vi "Unpack User Menu Selection.vi"(11 "UserMenuSelectionMsg In":refnum<class "UserMenuSelectionMsg.lvclass">) -> (0 "Item Path":string, 1 "Item Tag":string, 2 "Time":u32, 3 "MenuRef":refnum<k9>)   [LabVIEW 2015, in "ActorEvents.lvlib" / "UserMenuSelectionMsg.lvclass"]
doc: "<License>\nCopyright © 2017 Composed Systems, LLC | All rights reserved\nwww.composed.io\n\nAuthor: Ethan Stern <ethan.stern@composed.io>\n\nThis software is provided \"AS IS\" WITHOUT WARRANTIES, either express or implied, AND IS FOR EDUCATIONAL PURPOSES ONLY.\n</License>"
uses:
  UserMenuSelectionMsg.lvclass
  UserMenuSelectionMsg.lvclass/UserMenuSelectionMsg.ctl
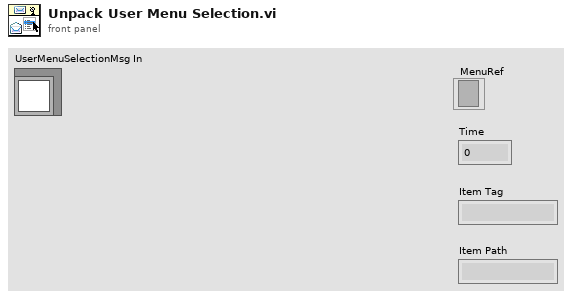
[diagram p1: front panel]
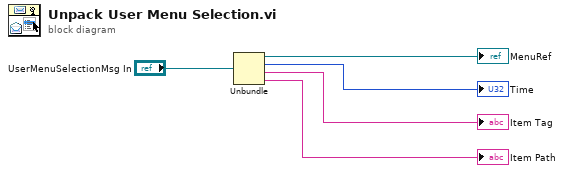
[diagram p0: block diagram]
diagram:
  n1 = Unbundle("UserMenuSelectionMsg In") -> (→"MenuRef":refnum<k9>, →"Time":u32, →"Item Tag":string, →"Item Path":string)
